vi "Clean Up.vi"(8 "error in (no error)":errorcluster, 11 "TDCManager":T1) -> (0 "error out":errorcluster, 3 "TDCManager out":T1)   [LabVIEW 2016, in "HPTDC Driver Library.lvlib"]
uses:
  HPTDC Driver Library.lvlib
  Typedefs/TDCManager.ctl
  C:/Users/CRT Controller/CRTC Labview Application/Source/HPTDC Driver Library Folder/Library files/hptdc_net4_3.7.0_x64.dll
  hptdc_net4_3.7.0_x64.dll
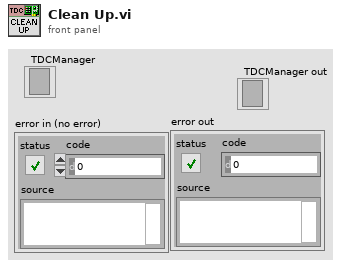
[diagram p1: front panel]
types:
  T1 = typedef "HPTDC Driver Library.lvlib/TDCManager.ctl" = refnum<k24>
  T2 = typedef "Semaphore RefNum" = refnum<k1>
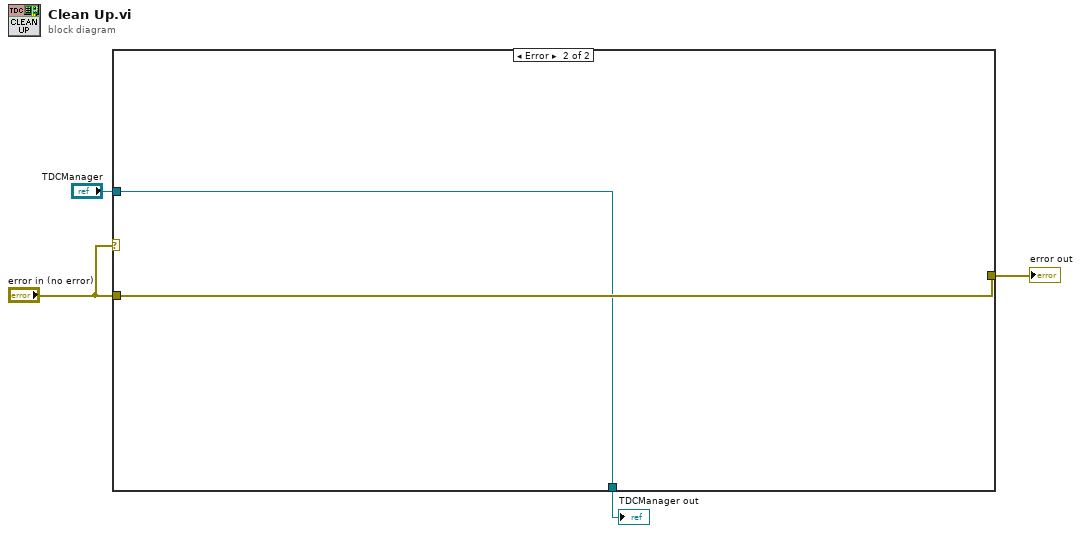
[diagram p0: block diagram]
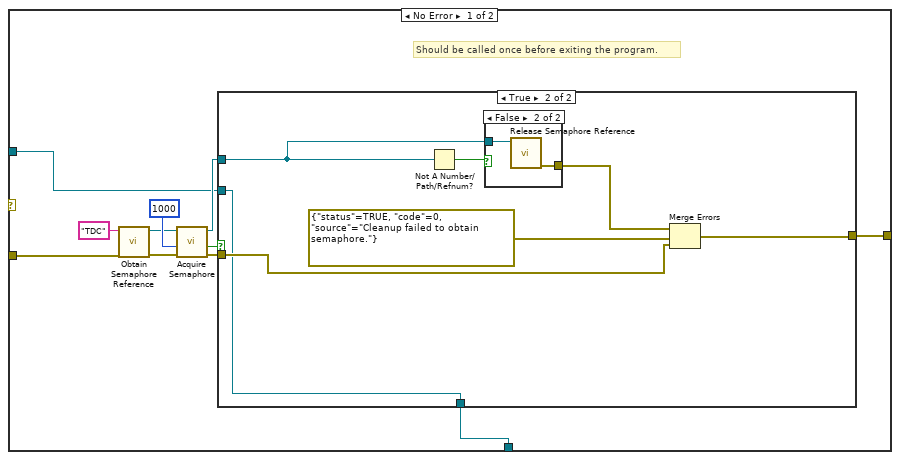
[diagram p2: hidden frame]
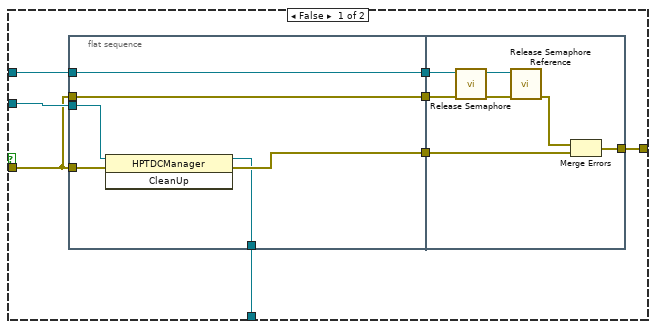
[diagram p3: hidden frame]
diagram:
  n1 = case shown="Error" "error in (no error)" {
    tunnel: "error in (no error)" -> [w8 w47]
    tunnel: [w7 w47] -> w4
    tunnel: "TDCManager" -> [w6 w46]
    tunnel: [w5 w46] -> w1
    frame No Error {
      # "Should be called once before exiting the program."
      n2 = call <vilib>:"Obtain Semaphore Reference.vi"("error in (no error)"=w8, "name (unnamed)"="TDC") -> ("error out"=w13:errorcluster, "semaphore"=w14:T2)  [unwired: 3 in, 1 out]
      n3 = call <vilib>:"Acquire Semaphore.vi"("error in (no error)"=w13, "ms timeout (-1)"=1000, "semaphore"=w14) -> ("error out"=w10:errorcluster, "timed out"=w11:bool, "semaphore out"=w9:T2)  [unwired: 2 in]
      n4 = case shown="True" w11 {
        tunnel: w6 -> [w23 w37]
        tunnel: w10 -> [w20 w39]
        tunnel: w9 -> [w18 w38]
        tunnel: [w17 w37] -> w5
        tunnel: [w16 w40] -> w7
        frame False {
          n5 = flat-sequence {
            tunnel: w20 -> [w29]
            tunnel: w23 -> [w28]
            tunnel: [w27] -> w22
            tunnel: w20 -> [w26]
            tunnel: [w26] -> w21
            tunnel: [w25] -> w19
            tunnel: w18 -> [w25]
            tunnel: [w24] -> w17
            tunnel: w22 -> [w36]
            tunnel: w21 -> [w33]
            tunnel: w19 -> [w31]
            tunnel: [w30] -> w16
            frame #0 {
              n6 = invoke class="HPTDCManager" method="CleanUp"(reference=w28, error in=w29) -> (reference out=w24:T1, error out=w27:errorcluster)  [unwired: 1 in, 1 out]
            }
            frame #1 {
              n7 = call <vilib>:"Release Semaphore.vi"("error in (no error)"=w33, "semaphore"=w31) -> ("error out"=w34:errorcluster, "semaphore out"=w35:T2)  [unwired: 4 in]
              n8 = call <vilib>:"Release Semaphore Reference.vi"("error in (no error)"=w34, "semaphore"=w35) -> ("error out"=w32:errorcluster)  [unwired: 8 in, 1 out]
              n9 = Merge Errors(w32, w36) -> (w30:errorcluster)
            }
          }
        }
        frame True {
          n10 = Not A Number/Path/Refnum?(number/path/refnum=w38) -> (NaN/Path/Refnum?=w43:bool)
          n11 = case shown="False" w43 {
            tunnel: [_ w45] -> w42
            tunnel: w38 -> [_ w44]
            frame True {
            }
            frame False {
              n12 = call <vilib>:"Release Semaphore Reference.vi"("semaphore"=w44) -> ("error out"=w45:errorcluster)  [unwired: 9 in, 1 out]
            }
          }
          n13 = Merge Errors(w42, errorcluster {"status"=TRUE, "code"=0, "source"="Cleanup failed to obtain semaphore."} ("error out"), w39) -> (w40:errorcluster)
        }
      }
    }
    frame Error {
    }
  }
  "error out" <- w4
  "TDCManager out" <- w1
